vi "Draw Rectangle (Greyscale).vi"(5 "Thickness (Default: 1)":i32=1, 6 "OpenCV Line Type (Default LINE_8)":T3=enum."LINE_8", 7 "Colour":u8=255, 8 "error in (no error)":errorcluster, 9 "Point B":T1, 10 "Point A":T1, 11 "Greyscale Image in":T2) -> (0 "error out":errorcluster, 3 "Greyscale Image":T2)   [LabVIEW 2020, in "image.lvlib"]
doc: "Draw a rectangle based on the two corner points given."
uses:
  image.lvlib
  Line Type.ctl
  common/Image Point (Integer).ctl
  Greyscale Image.ctl
  7e6fb015-3761-4366-a0a7-e436eb229083.vi
  <vilib>/Utility/error.llb/Error Cluster From Error Code.vi
  common/common.lvlib
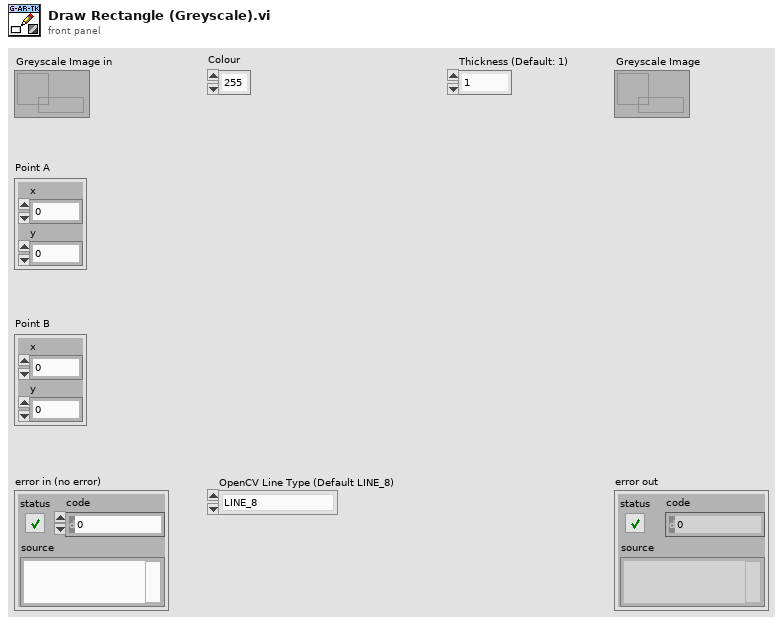
[diagram p1: front panel]
types:
  T1 = typedef "common.lvlib/Image Point (Integer).ctl" = cluster{"x":i32, "y":i32}
  T2 = typedef "image.lvlib/Greyscale Image.ctl" = refnum<data-value>
  T3 = typedef "image.lvlib/Line Type.ctl" = enum8{"FILLED", "LINE_4", "LINE_8", "LINE_AA"}
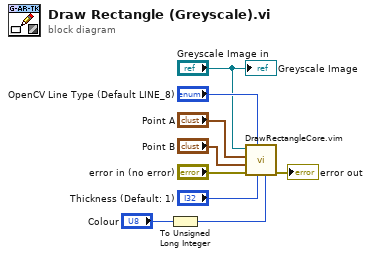
[diagram p0: block diagram]
diagram:
  n1 = To Unsigned Long Integer(number="Colour") -> (unsigned 32bit integer=w2:u32)
  n2 = call "DrawRectangleCore.vim"("Colour"=w2, "Thickness"="Thickness (Default: 1)", "OpenCV Line Type"="OpenCV Line Type (Default LINE_8)", "error in (no error)"="error in (no error)", "Point B"="Point B", "Point A"="Point A", "Src"="Greyscale Image in") -> ("error out"=→"error out":errorcluster)  [unwired: 4 in]
  "Greyscale Image" <- "Greyscale Image in"
